vi "WriteCamCal.vi"   [LabVIEW 2016]
uses:
  <vilib>/Rock Robotics/Network Tables/NT Read Number.vi
  <vilib>/Utility/config.llb/Write Key (Double).vi
  <vilib>/Utility/config.llb/NI_LVConfig.lvlib
types:
  T1 = typedef "NI_LVConfig.lvlib/Config Data RefNum.ctl" = refnum<k1>
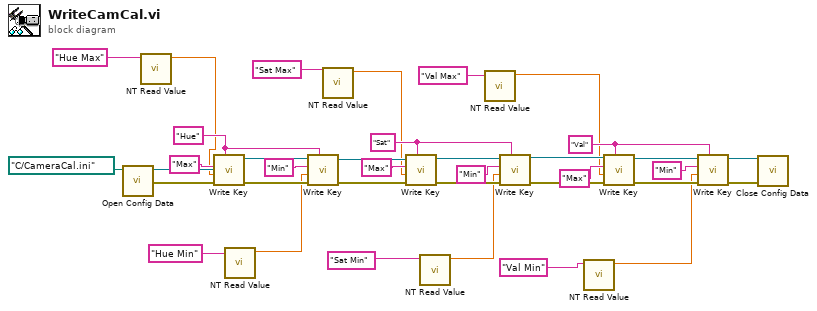
[diagram p0: block diagram]
diagram:
  w23 = "Val" ("section")
  w24 = "Sat" ("section")
  w36 = "Hue" ("section")
  n1 = call <vilib>:"Open Config Data.vi"("configuration file path"=path "C:/CameraCal.ini") -> ("error out"=w31:errorcluster, "refnum"=w30:T1)  [unwired: 8 in, 1 out]
  n2 = call-poly <vilib>:"NT Read Value.vi"("Name"="Hue Max" ("section")) -> ("Numeric"=w6:dbl)  [unwired: 9 in, 1 out]
  n3 = call-poly <vilib>:"Write Key.vi"("section"=w36, "error in (no error)"=w31, "value"=w6, "key"="Max", "refnum"=w30) -> ("error out"=w35:errorcluster, "refnum out"=w34:T1)  [unwired: 4 in, 1 out]
  n4 = call-poly <vilib>:"NT Read Value.vi"("Name"="Hue Min" ("section")) -> ("Numeric"=w5:dbl)  [unwired: 9 in, 1 out]
  n5 = call-poly <vilib>:"Write Key.vi"("section"=w36, "error in (no error)"=w35, "value"=w5, "key"="Min", "refnum"=w34) -> ("error out"=w17:errorcluster, "refnum out"=w18:T1)  [unwired: 4 in, 1 out]
  n6 = call-poly <vilib>:"NT Read Value.vi"("Name"="Sat Max" ("section")) -> ("Numeric"=w4:dbl)  [unwired: 9 in, 1 out]
  n7 = call-poly <vilib>:"Write Key.vi"("section"=w24, "error in (no error)"=w17, "value"=w4, "key"="Max", "refnum"=w18) -> ("error out"=w25:errorcluster, "refnum out"=w26:T1)  [unwired: 4 in, 1 out]
  n8 = call-poly <vilib>:"NT Read Value.vi"("Name"="Sat Min" ("section")) -> ("Numeric"=w3:dbl)  [unwired: 9 in, 1 out]
  n9 = call-poly <vilib>:"NT Read Value.vi"("Name"="Val Max" ("section")) -> ("Numeric"=w2:dbl)  [unwired: 9 in, 1 out]
  n10 = call-poly <vilib>:"Write Key.vi"("section"=w24, "error in (no error)"=w25, "value"=w3, "key"="Min", "refnum"=w26) -> ("error out"=w15:errorcluster, "refnum out"=w16:T1)  [unwired: 4 in, 1 out]
  n11 = call-poly <vilib>:"NT Read Value.vi"("Name"="Val Min" ("section")) -> ("Numeric"=w1:dbl)  [unwired: 9 in, 1 out]
  n12 = call-poly <vilib>:"Write Key.vi"("section"=w23, "error in (no error)"=w15, "value"=w2, "key"="Max", "refnum"=w16) -> ("error out"=w22:errorcluster, "refnum out"=w21:T1)  [unwired: 4 in, 1 out]
  n13 = call-poly <vilib>:"Write Key.vi"("section"=w23, "error in (no error)"=w22, "value"=w1, "key"="Min", "refnum"=w21) -> ("error out"=w14:errorcluster, "refnum out"=w13:T1)  [unwired: 4 in, 1 out]
  n14 = call <vilib>:"Close Config Data.vi"("error in (no error)"=w14, "refnum"=w13) -> ()  [unwired: 8 in, 2 out]
